vi "Update Delay.vi"(7 "BME_DG_System":refnum<class "BME_DG_System.lvclass">, 8 "error in (no error)":errorcluster, 10 "Chnl A":refnum<class "BME_DG_Chnl.lvclass">, 11 "Chnl2Change":refnum<class "BME_DG_Chnl.lvclass">) -> (0 "error out":errorcluster, 5 "BME_DG_System out":refnum<class "BME_DG_System.lvclass">)   [LabVIEW 2009, in "POLARIS BME DG.lvlib" / "BME_DG_Chnl.lvclass"]
uses:
  BME_DG_Chnl.lvclass
  BME_DG_System/BME_DG_System.lvclass
  BME_DG_Chnl.lvclass/BME_DG_Chnl.ctl
  <vilib>/gmath/NI_Gmath.lvlib
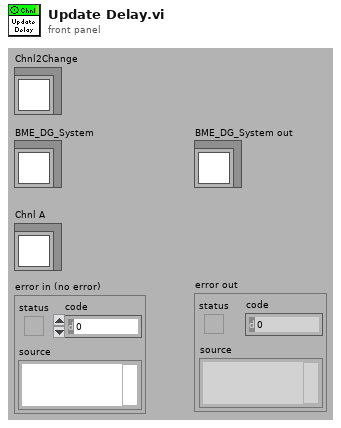
[diagram p1: front panel]
types:
  T1 = typedef "POLARIS BME DG.lvlib/ChnlSettings.ctl" = cluster{" Delay (µs)":dbl, "On? (false)":bool, "PositiveVoltage?":bool, "50OhmTerminated? ":bool, "25OhmOutput?":bool}
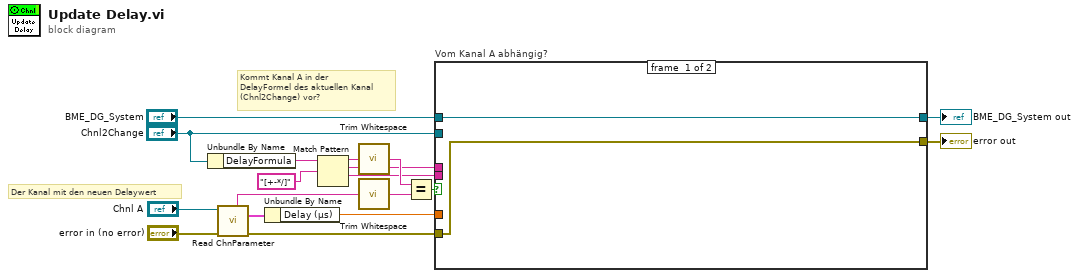
[diagram p0: block diagram]
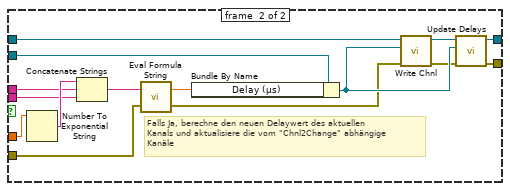
[diagram p2: hidden frame]
diagram:
  # "Kommt Kanal A in der \nDelayFormel des aktuellen Kanal\n(Chnl2Change) vor?"
  # "Der Kanal mit den neuen Delaywert"
  n1 = Unbundle By Name("Chnl2Change") -> ("DelayFormula"=w14:string)
  n2 = call-dynamic "Read ChnParameter.vi"("error in (no error)"="error in (no error)", "BME_DG_Chnl in"="Chnl A") -> ("error out"=w1:errorcluster, "ChnParemater"=w3:T1, "Name"=w4:string)  [unwired: 4 in, 3 out]
  n3 = Unbundle By Name(w3) -> ("Delay (µs)"=w2:dbl)
  n4 = Match Pattern(string=w14, regular expression="[+-*/]") -> (before substring=w16:string, match substring=w9:string, after substring=w8:string)  [unwired: 1 in, 1 out]
  n5 = call <vilib>:"Trim Whitespace.vi"("string"=w16) -> ("trimmed string"=w13:string)  [unwired: 1 in]
  n6 = call <vilib>:"Trim Whitespace.vi"("string"=w4) -> ("trimmed string"=w12:string)  [unwired: 1 in]
  n7 = Equal?(x=w13, y=w12) -> (x = y?=w11:bool)
  n8 = case "Vom Kanal A abhängig?" shown="True" w11 {
    tunnel: [w19 w35] -> w18
    tunnel: "Chnl2Change" -> [_ w34]
    tunnel: "BME_DG_System" -> [w20 w25]
    tunnel: w2 -> [_ w32]
    tunnel: w9 -> [_ w30]
    tunnel: w8 -> [_ w29]
    tunnel: [w20 w27] -> w7
    tunnel: w1 -> [w19 w26]
    frame #0 {
    }
    frame #1 {
      # "Falls Ja, berechne den neuen Delaywert des aktuellen\nKanals und aktualisiere die vom \"Chnl2Change\" abhängige\nKanäle"
      n9 = Number To Exponential String(number=w32) -> (E-format string=w31:string)  [unwired: 3 in]
      n10 = Concatenate Strings(w31, w30, w29) -> (w33:string)
      n11 = call <vilib>:"Eval Formula String.vi"("error in (no error)"=w26, "formula"=w33) -> ("error out"=w22:errorcluster, "y value"=w28:dbl)
      n12 = Bundle By Name(cluster=w34, "Delay (µs)"=w28) -> (w23:refnum<class "BME_DG_Chnl.lvclass">)
      n13 = call "Write Chnl.vi"("error in (no error)"=w22, "BME_DG_Chnl.lvclass"=w23, "BME_DG_System in"=w25) -> ("error out"=w21:errorcluster, "BME_DG_System out"=w24:refnum<class "BME_DG_System.lvclass">)  [unwired: 7 in]
      n14 = call "Update Delays.vi"("error in (no error)"=w21, "BME_DG_Chnl in"=w23, "BME_DG_System in"=w24) -> ("error out"=w35:errorcluster, "BME_DG_System out"=w27:refnum<class "BME_DG_System.lvclass">)  [unwired: 7 in]
    }
  }
  "error out" <- w18
  "BME_DG_System out" <- w7
